vi "Find Colleague.vi"(0 "reference in":refnum<class "Mediator.lvclass">, 2 "Name":string, 5 "error in (no error)":errorcluster) -> (14 "reference out":refnum<class "Mediator.lvclass">, 16 "Colleague.lvclass":refnum<class "Colleague.lvclass">, 19 "error out":errorcluster)   [LabVIEW 2013, in "Mediator.lvclass"]
uses:
  Mediator.lvclass
  Colleague_class/Colleague.lvclass
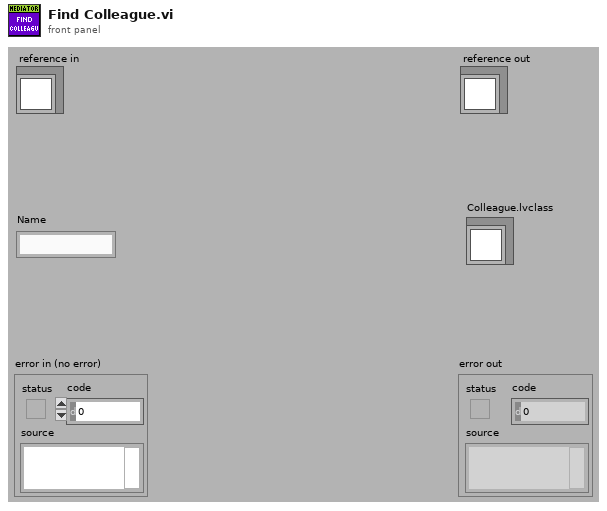
[diagram p1: front panel]
types:
  T1 = typedef "Mediator.lvclass/ObjectAttributes.ctl" = cluster{"Colleague":refnum<class "Colleague.lvclass">[], "Name":string[]}
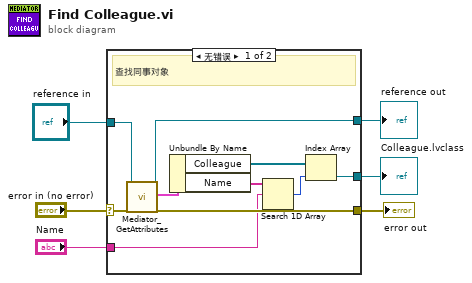
[diagram p0: block diagram]
diagram:
  n1 = case shown="无错误" "error in (no error)" {
    selector: "error in (no error)" -> [w16 w18]
    tunnel: [w15 w18] -> w5
    tunnel: [w14 w17] -> w3
    tunnel: "reference in" -> [w12 w17]
    tunnel: "Name" -> [w11 _]
    tunnel: [w7 _] -> w1
    frame No Error {
      # "查找同事对象"
      n2 = call "Mediator_GetAttributes.vi"("reference in"=w12, "error in (no error)"=w16) -> ("reference out"=w14:refnum<class "Mediator.lvclass">, "attributes"=w13:T1, "error out"=w15:errorcluster)  [unwired: 14 in, 1 out]
      n3 = Unbundle By Name(w13) -> ("Colleague"=w9:refnum<class "Colleague.lvclass">[], "Name"=w10:string[])
      n4 = Search 1D Array(1D array=w10, element=w11) -> (index of element=w8:i32)  [unwired: 1 in]
      n5 = Index Array(array=w9, index=w8) -> (element=w7:refnum<class "Colleague.lvclass">)
    }
    frame Error {
    }
  }
  "error out" <- w5
  "reference out" <- w3
  "Colleague.lvclass" <- w1
